vi "ni579x Configure LO Frequency.vi"(0 "Register Bus":refnum<class "ni579x Register Bus v1 Host.lvclass">=refnum, 1 "scope":string(combo)="LO1", 5 "frequency [Hz]":dbl format="%#_6p", 11 "Error In":errorcluster) -> (4 "Register Bus (out)":refnum<class "ni579x Register Bus v1 Host.lvclass">, 6 "coerced frequency [Hz]":dbl format="%#_6p", 15 "Error Out":errorcluster)   [LabVIEW 2013]
uses:
  <instrlib>/ni579x/Register Bus/v1/Host/ni579x Register Bus v1 Host.lvclass
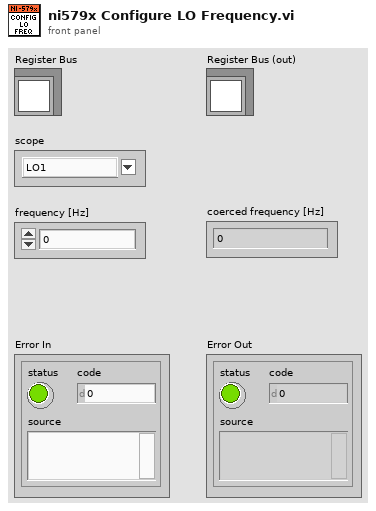
[diagram p1: front panel]
types:
  T1 = typedef "ni579x FAM Register Operation.ctl" = cluster{"FAM Register Offset":T2, "Address":u32, "Write (T)/Read (F)":bool, "Write Data":u32}
  T2 = typedef "ni579x FAM Register Offset.ctl" = u8
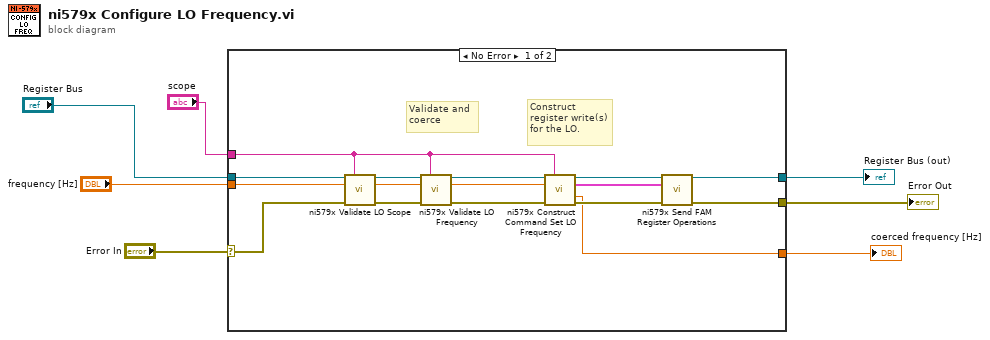
[diagram p0: block diagram]
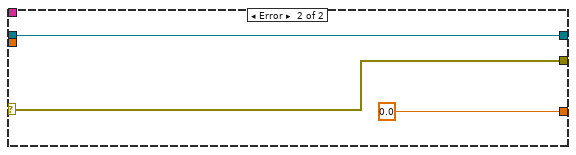
[diagram p2: hidden frame]
diagram:
  n1 = case shown="No Error" "Error In" {
    selector: "Error In" -> [w14 w25]
    tunnel: [w15 w25] -> w6
    tunnel: "Register Bus" -> [w12 w24]
    tunnel: "frequency [Hz]" -> [w22 _]
    tunnel: [w16 w24] -> w3
    tunnel: [w8 0.0 ("coerced attenuation [dB]")] -> w2
    tunnel: "scope" -> [w10 _]
    frame No Error {
      # "Construct\nregister write(s)\nfor the LO."
      # "Validate and \ncoerce"
      n2 = call <instrlib>:"ni579x Validate LO Scope.vi"("Register Bus"=w12, "scope"=w10, "Error In"=w14) -> ("Register Bus (out)"=w11:refnum<class "ni579x Register Bus v1 Host.lvclass">, "Error Out"=w13:errorcluster)  [unwired: 11 in]
      n3 = call <instrlib>:"ni579x Validate LO Frequency.vi"("Register Bus"=w11, "scope"=w10, "frequency [Hz]"=w22, "Error In"=w13) -> ("Register Bus (out)"=w20:refnum<class "ni579x Register Bus v1 Host.lvclass">, "coerced frequency [Hz]"=w9:dbl, "Error Out"=w21:errorcluster)  [unwired: 9 in]
      n4 = call <instrlib>:"ni579x Construct Command Set LO Frequency.vi"("Register Bus"=w20, "scope"=w10, "frequency [Hz]"=w9, "Error In"=w21) -> ("Register Bus (out)"=w19:refnum<class "ni579x Register Bus v1 Host.lvclass">, "FAM Register Operations"=w17:T1[], "coerced frequency [Hz]"=w8:dbl, "Error Out"=w18:errorcluster)  [unwired: 8 in]
      n5 = call <instrlib>:"ni579x Send FAM Register Operations.vi"("Register Bus"=w19, "FAM Register Operations"=w17, "Error In"=w18) -> ("Register Bus (out)"=w16:refnum<class "ni579x Register Bus v1 Host.lvclass">, "Error Out"=w15:errorcluster)  [unwired: 10 in, 1 out]
    }
    frame Error {
    }
  }
  "Register Bus (out)" <- w3
  "Error Out" <- w6
  "coerced frequency [Hz]" <- w2
